vi "Write Base U64.vi"(4 "timestamps":timestamp[](array[numeric]), 6 "index_channel":u32, 8 "error in":errorcluster, 9 "data":u64[][](array[numeric]), 10 "channels":u32[](array[numeric]), 11 "Writer":refnum<class "Synnax Writer.lvclass">) -> (0 "error out":errorcluster, 3 "Writer Out":refnum<class "Synnax Writer.lvclass">)   [LabVIEW 2026, in "synnax_lib.lvlib" / "Synnax Writer.lvclass"]
doc: "SYNNAX_EXPORT int32_t synnax_writer_write(\n SynnaxWriter writer,\n uint32_t channel,\n const double *data,\n uint64_t sample_count,\n SynnaxError err\n);"
uses:
  Synnax Writer.lvclass
  Synnax Writer.lvclass/Synnax Writer.ctl
  <vilib>/Utility/error.llb/Error Cluster From Error Code.vi
  synnax_lib.lvlib
  synnax_clib.dll
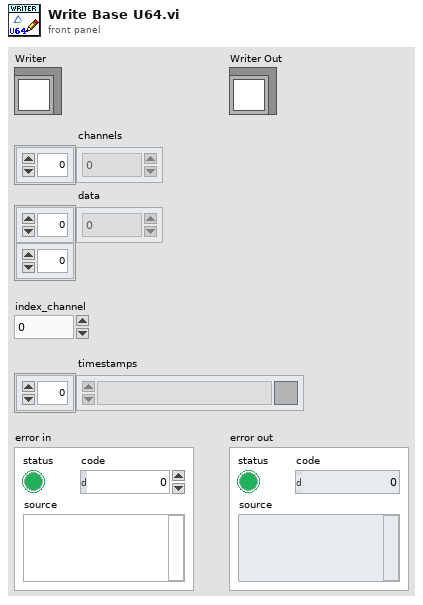
[diagram p1: front panel]
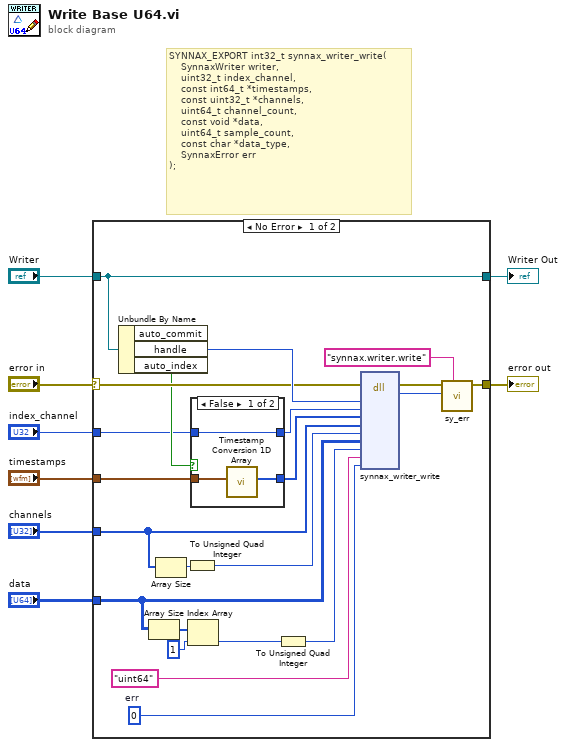
[diagram p0: block diagram]
diagram:
  # "SYNNAX_EXPORT int32_t synnax_writer_write(\n    SynnaxWriter writer,\n    uint32_t index_channel,\n    const int64_t *timestamps,\n    const uint32_t *channels,\n    uint64_t channel_count,\n    const void *data,\n    uint64_t sample_count,\n    const char *data_type,\n    SynnaxError err\n);"
  n1 = case shown="No Error" "error in" {
    selector: "error in" -> [w16 w35]
    tunnel: "index_channel" -> [w14 _]
    tunnel: [w12 w35] -> w7
    tunnel: "channels" -> [w25 _]
    tunnel: "data" -> [w23 _]
    tunnel: "timestamps" -> [w19 _]
    tunnel: "Writer" -> [w11 w34]
    tunnel: [w11 w34] -> w1
    frame No Error {
      w10 = u64 0  # err
      n2 = Unbundle By Name(w11) -> ("handle"=w17:u64, "auto_index"=w15:bool)  [unwired: 1 out]
      n3 = Array Size(array=w23) -> (size(s)=w22:i32[])
      n4 = Array Size(array=w25) -> (size(s)=w27:i32)
      n5 = To Unsigned Quad Integer(1:w27) -> (0:w26:u64)
      n6 = Index Array(array=w22, index=1) -> (element=w21:i32)
      n7 = case shown="False" w15 {
        tunnel: w19 -> [w33 _]
        tunnel: [w32 _] -> w18
        tunnel: w14 -> [w31 _]
        tunnel: [w31 _] -> w13
        frame False {
          n8 = call "Timestamp Conversion 1D Array.vi"("timestamps"=w33) -> ("timestamps (ns)"=w32:i64[])  [unwired: 9 in]
        }
        frame True {
        }
      }
      n9 = To Unsigned Quad Integer(1:w21) -> (0:w24:u64)
      n10 = dll-call lib="C/synnax/client/lv/synnax_clib.dll" fn="synnax_writer_write"(error in=w16, "writer"=w17, "index_channel"=w13, "timestamps"=w18, "channels"=w25, "channel_count"=w26, "data"=w23, "sample_count"=w24, "data_type"="uint64", "err"=w10) -> (error out=w30:errorcluster, "return type"=w29:i32)  [unwired: 11 in, 1 out]
      n11 = call "sy_err.vi"("source"="synnax.writer.write", "error code"=w29, "error in (no error)"=w30) -> ("error out"=w12:errorcluster)  [unwired: 8 in]
    }
    frame Error {
    }
  }
  "error out" <- w7
  "Writer Out" <- w1
